vi "PSUN8731A-CTRLv2.vi"() -> ()   [LabVIEW 2017]
uses:
  Keysight N8731A conversion/Keysight N8900 Series.lvlib
panel:
  in  "Visible":bool
  in  "End Program":bool
  in  "PSU\nVoltage":bool caption="Keithley\nVoltage"
  in  "Sweep":bool caption="Constant"
  in  "OV protection":bool
  in  "Filename":string caption="Leave empty to discard data."
  out "Sweeping Back":bool
  in  "OC protection":bool
  in  "OV Value (10V)":dbl=10.0 min=0.5 max=10.0
  in  "Start Sweep":bool
  in  "Stop Sweep":bool
  in  "Sweep Controller":enum32{"CC Sweep", "Free Control", "VC Sweep"}(tab)
  in  "Voltage Limit [V]":dbl=8.0 min=0.0 max=8.0
  in  "Time Delay [s]":dbl=0.15
  in  "Step Size [A]":dbl=5.0 min=0.0 max=400.0
  in  "Start Current [A]":dbl min=0.0 max=400.0
  in  "End Current [A]":dbl=50.0 min=0.0 max=400.0
  out "Approx Run Time [min]":dbl
  in  "Current Limit [A]":dbl=150.0 min=0.0 max=400.0
  in  "Time Delay [s]":dbl=0.15 min=0.0
  in  "Step Size [mV]":dbl=10.0 min=0.0
  in  "Start Voltage [V]":dbl min=0.0 max=8.0
  in  "End Voltage[V]":dbl=0.1 min=0.0 max=8.0
  out "Approx Run Time [min]":dbl
  in  "VISA resource name":refnum<visa-resource-name>
  out "XY Graph":cluster{dbl[], dbl[]}(graph)
  # "Requires the subVIs in the \"Controller subVIs\" folder to function."
  # "\"Stop Sweep\" will immediately begin sweeping back to 0."
  # "Correct VISA option: TCPIP0::A-N8731A-8956R.local::inst0::INSTR\nfor lab computer or N8731APSU on the EPR computer."
  # "Sweep type will be automatically chosen according to open tab"
  # "Parameters may be\nedited before starting\nsweep"
  # "In case of errors, first check whether OVP or\nOCP has been triggered, or if parameters are \noutside allowed range. Currently leading causes\nof crashes."
  # "OCP not functional with CC\nsweeps, reason thus far unknown.\nSolution: disable OCP if safe."
  # "Data will be saved in .txt format, further analysis should be done on a\nseparate platform such as Gnuplot."
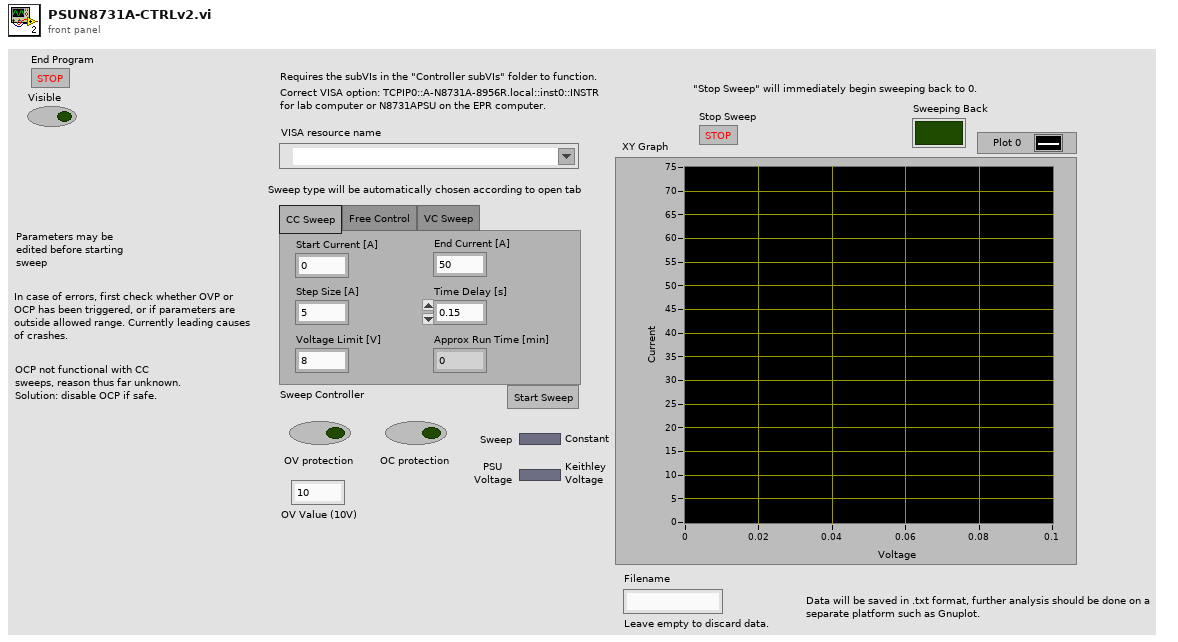
[diagram p1: front panel]
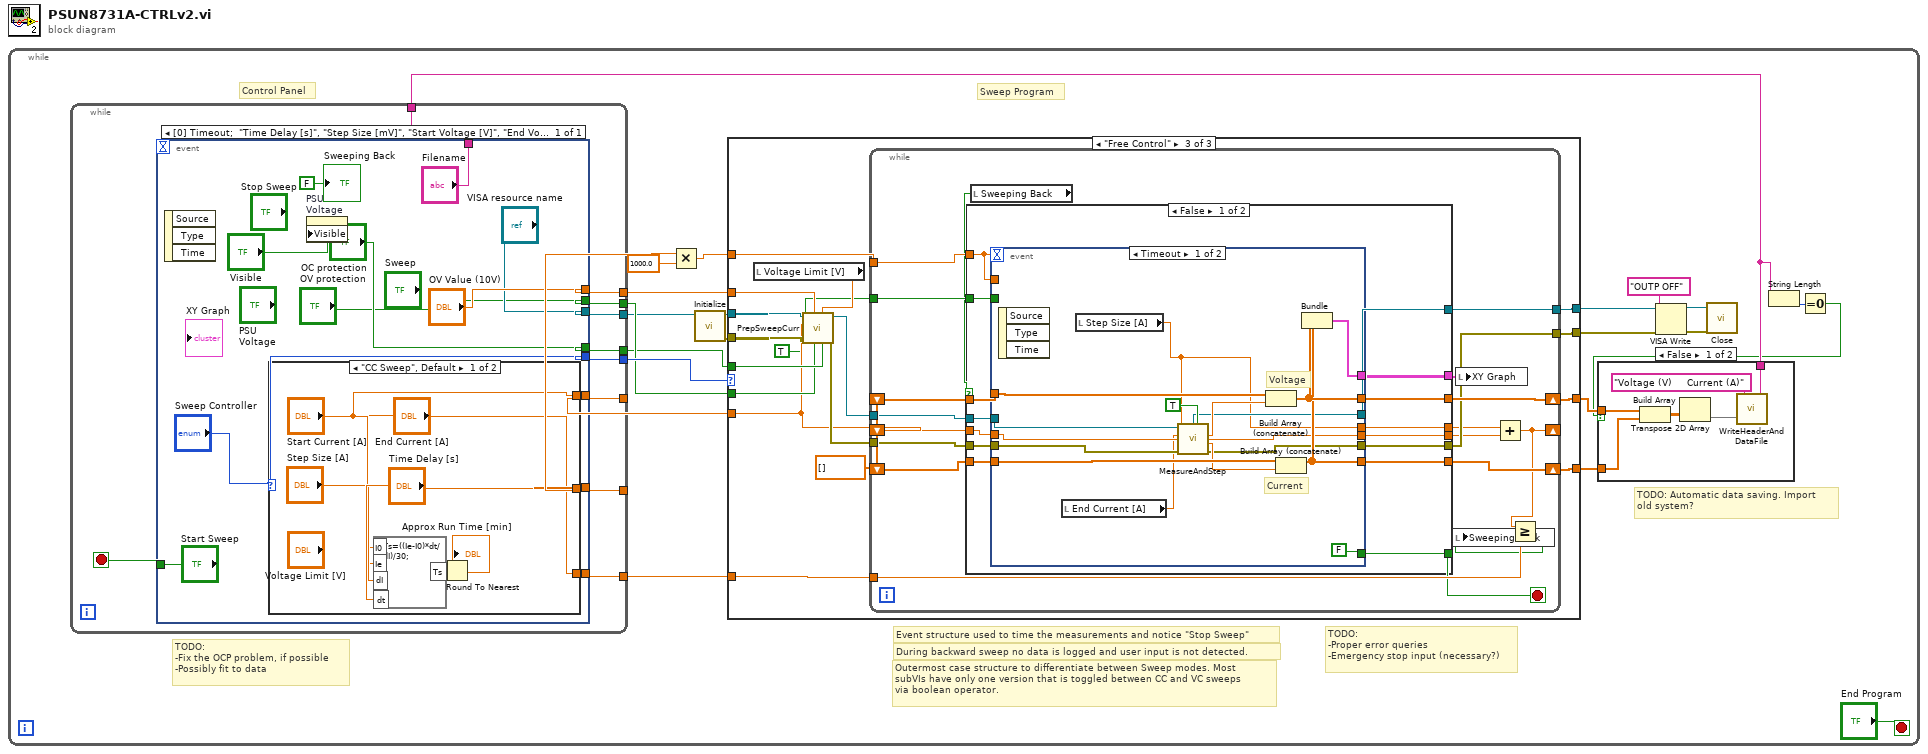
[diagram p0: block diagram]
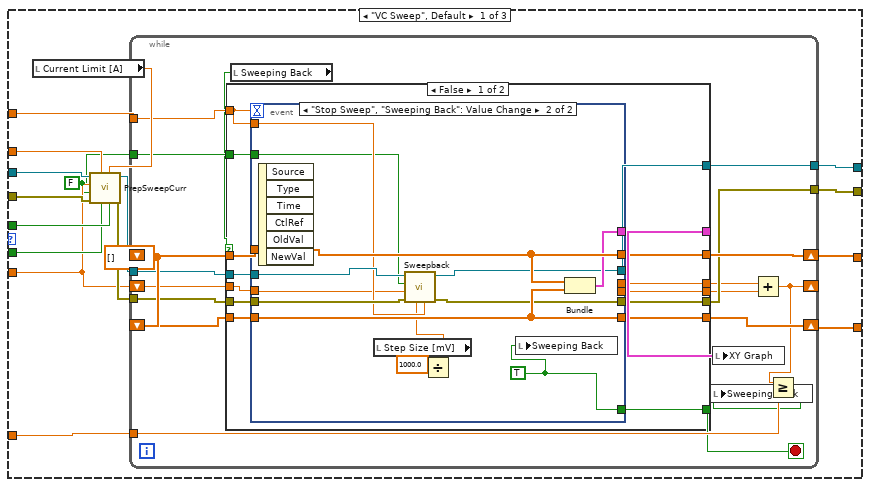
[diagram p3: hidden frame]
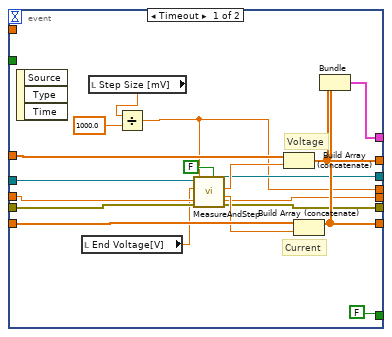
[diagram p4: hidden frame]
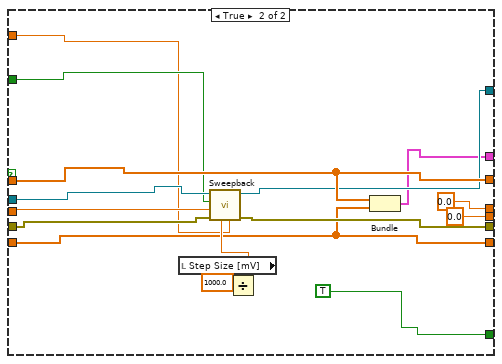
[diagram p5: hidden frame]
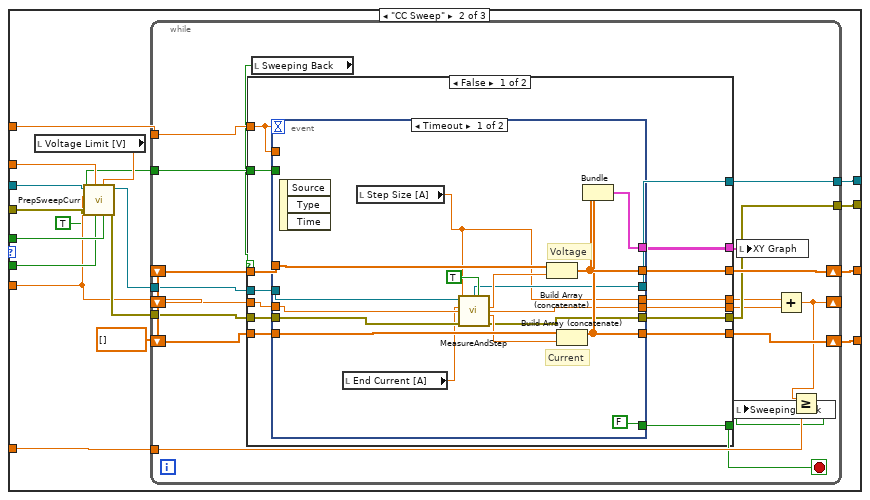
[diagram p6: hidden frame]
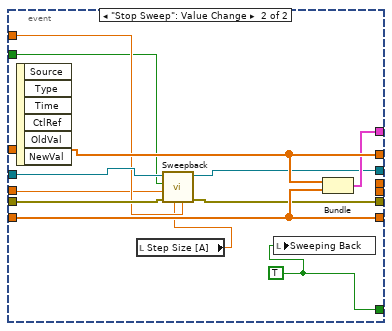
[diagram p7: hidden frame]
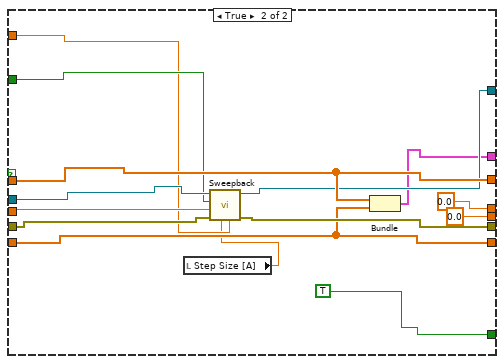
[diagram p8: hidden frame]
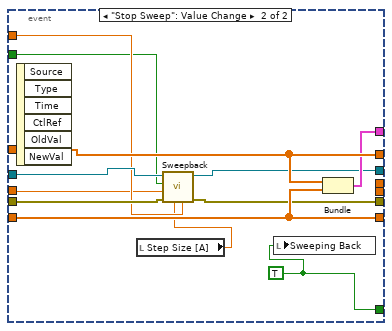
[diagram p9: hidden frame]
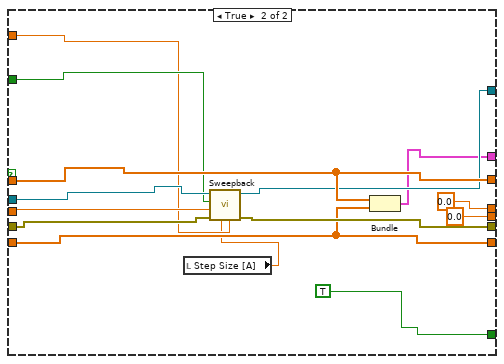
[diagram p10: hidden frame]
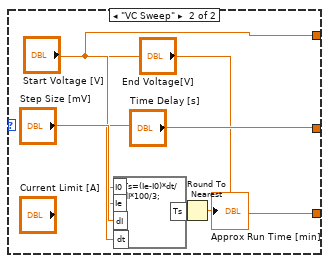
[diagram p11: hidden frame]
diagram:
  n1 = while {
    stop <- "End Program" stop-if-true
    # "TODO: \n-Proper error queries\n-Emergency stop input (necessary?)"
    # "TODO: Automatic data saving. Import\nold system?"
    # "TODO: \n-Fix the OCP problem, if possible\n-Possibly fit to data"
    # "Outermost case structure to differentiate between Sweep modes. Most\nsubVIs have only one version that is toggled between CC and VC sweeps\nvia boolean operator."
    # "During backward sweep no data is logged and user input is not detected."
    # "Event structure used to time the measurements and notice \"Stop Sweep\""
    # "Sweep Program"
    # "Control Panel"
    n2 = while {
      tunnel: [w324] -> w11
      tunnel: [w322] -> w23
      tunnel: [w321] -> w22
      tunnel: [w320] -> w8
      tunnel: [w315] -> w19
      tunnel: [w319] -> w18
      tunnel: [w318] -> w17
      tunnel: [w317] -> w7
      tunnel: [w316] -> w4
      stop <- w323 stop-if-true
      n3 = event shown="[0] Timeout;  \"Time Delay [s]\", \"Step Size [mV]\", \"Start Voltage [V]\", \"End Voltage[V]\", \"XY Graph\", \"VISA resource name\", \"Sweep Controller\", \"End Current [A]\", \"Stop Sweep\", \"Start Current [A]\", \"Step Size [A]\", \"Time Delay [s]\", \"Current Limit [A]\", \"Voltage Limit [V]\", \"Start Sweep\", \"Approx Run Time [min]\", \"Approx Run Time [min]\", \"OV Value (10V)\", \"OC protection\", \"Sweeping Back\", \"Filename\", \"OV protection\", \"PSU Voltage\": Value Change" {
        selector: _ -> [_]
        dyn-events: _ -> [_]
        timeout: _ -> [_]
        tunnel: [w336] -> w324
        tunnel: ["Start Sweep"] -> w323
        tunnel: [w334] -> w322
        tunnel: ["Sweep Controller"] -> w321
        tunnel: ["OC protection"] -> w320
        tunnel: ["OV Value (10V)"] -> w319
        tunnel: [w330] -> w318
        tunnel: ["VISA resource name"] -> w317
        tunnel: ["Filename"] -> w316
        tunnel: ["OV protection"] -> w315
        event Timeout; "Time Delay [s]", "Step Size [mV]", "Start Voltage [V]", "End Voltage[V]", "XY Graph", "VISA resource name", "Sweep Controller", "End Current [A]", "Stop Sweep", "Start Current [A]", "Step Size [A]", "Time Delay [s]", "Current Limit [A]", "Voltage Limit [V]", "Start Sweep", "Approx Run Time [min]", "Approx Run Time [min]", "OV Value (10V)", "OC protection", "Sweeping Back", "Filename", "OV protection", "PSU\nVoltage": Value Change {
          n4 = event-data() -> ()  [unwired: 1 in, 3 out]
          n5 = case shown="\"CC Sweep\", Default" "Sweep Controller" {
            tunnel: ["Time Delay [s]" "Time Delay [s]"] -> w336
            tunnel: ["Start Current [A]" "Start Voltage [V]"] -> w334
            tunnel: ["End Current [A]" "End Voltage[V]"] -> w330
            frame "CC Sweep", Default {
              n6 = formula code="Ts=((Ie-I0)*dt/dI)/30;"("I0"="Start Current [A]", "Ie"="End Current [A]", "dI"="Step Size [A]", "dt"="Time Delay [s]") -> ("Ts"=w340:dbl)
              n7 = Round To Nearest(number=w340) -> (nearest integer value=→"Approx Run Time [min]":dbl)
            }
            frame "VC Sweep" {
              n8 = formula code="Ts=(Ie-I0)*dt/dI*100/3;"("I0"="Start Voltage [V]", "Ie"="End Voltage[V]", "dI"="Step Size [mV]", "dt"="Time Delay [s]") -> ("Ts"=w346:dbl)
              n9 = Round To Nearest(number=w346) -> (nearest integer value=→"Approx Run Time [min]":dbl)
            }
          }
          n10 = property on="PSU\nVoltage" class="Bool (strict)"("Visible"="Visible") -> ()  [unwired: 2 in, 2 out]
          "Sweeping Back" <- FALSE ("Sweeping Back")
        }
      }
    }
    n11 = Multiply(x=w11, y=1000.0) -> (x*y=w10:dbl)
    n12 = call "Initialize.vi"("VISA resource name"=w7) -> ("error out"=w21:errorcluster, "VISA resource name out"=w20:refnum<visa-resource-name>)  [unwired: 9 in]
    n13 = case shown="\"Free Control\"" w22 {
      tunnel: w10 -> [w46 w145 w238]
      tunnel: w23 -> [w35 w134 w227]
      tunnel: w21 -> [w45 w144 w237]
      tunnel: w20 -> [w44 w143 w236]
      tunnel: [w41 w140 w233] -> w15
      tunnel: [w40 w139 w232] -> w16
      tunnel: w8 -> [w39 w138 w231]
      tunnel: w19 -> [w38 w137 w230]
      tunnel: w18 -> [w37 w136 w229]
      tunnel: w17 -> [w34 w133 w226]
      tunnel: [w31 w130 w223] -> w6
      tunnel: [w30 w129 w222] -> w5
      frame "VC Sweep", Default {
        w32 = dbl[] []
        w33 = FALSE ("CC (1)/VC (0)")
        n14 = local read "Current Limit [A]"() -> (w36:dbl)
        n15 = call "PrepSweepCurr.vi"("OC protection"=w39, "Voltage/Current Limit (0V/A)"=w36, "OV protection"=w38, "OV Value (10V)"=w37, "error in (no error)"=w45, "CC (1)/VC (0)"=w33, "Start Current/Voltage (0 A/V)"=w35, "VISA resource name"=w44) -> ("error out"=w42:errorcluster, "VISA resource name out"=w43:refnum<visa-resource-name>)  [unwired: 2 in]
        n16 = while {
          tunnel: w46 -> [w52]
          shift-right: [w65] -> w31
          shift-left: w32 -> [w63]
          shift-right: [w64] -> w30
          shift-left: w32 -> [w62]
          tunnel: w43 -> [w61]
          tunnel: w42 -> [w60]
          tunnel: [w59] -> w41
          tunnel: [w58] -> w40
          shift-right: [w55] -> _
          shift-left: w35 -> [w50]
          tunnel: w34 -> [w53]
          tunnel: w33 -> [w51]
          stop <- w49 stop-if-true
          n17 = local read "Sweeping Back"() -> (w48:bool)
          n18 = case shown="False" w48 {
            tunnel: [w80 w121] -> w65
            tunnel: [w79 w117] -> w64
            tunnel: w63 -> [w78 w121]
            tunnel: w62 -> [w77 w117]
            tunnel: w61 -> [w76 w122]
            tunnel: w60 -> [w75 w124]
            tunnel: [w74 w120] -> w59
            tunnel: [w73 w118] -> w58
            tunnel: [w72 0.0 ("Start Voltage [V]")] -> w57
            tunnel: [w71 w119] -> w56
            tunnel: [w70 0.0] -> w54
            tunnel: w52 -> [w69 w115]
            tunnel: w51 -> [w68 w116]
            tunnel: w50 -> [w67 w123]
            tunnel: [w66 TRUE] -> w49
            frame False {
              n19 = event shown="[1] \"Stop Sweep\", \"Sweeping Back\": Value Change" {
                selector: _ -> [_ _]
                dyn-events: _ -> [_ _]
                timeout: w69 -> [_ _]
                tunnel: [w98 w110] -> w71
                tunnel: [w97 w112] -> w80
                tunnel: [w96 w111] -> w79
                tunnel: w78 -> [w95 w112]
                tunnel: w77 -> [w94 w111]
                tunnel: [FALSE w99] -> w66
                tunnel: w76 -> [w87 w109]
                tunnel: w75 -> [w86 w107]
                tunnel: [w88 w106] -> w73
                tunnel: [w89 w108] -> w74
                tunnel: w67 -> [w85 w100]
                tunnel: [w85 _] -> w72
                tunnel: [w82 _] -> w70
                tunnel: w69 -> [_ w105]
                tunnel: w68 -> [_ w101]
                event Timeout {
                  # "Current"
                  # "Voltage"
                  n20 = event-data() -> ()  [unwired: 1 in, 3 out]
                  n21 = local read "End Voltage[V]"() -> (w81:dbl)
                  n22 = local read "Step Size [mV]"() -> (w84:dbl)
                  n23 = Divide(x=w84, y=1000.0) -> (x/y=w82:dbl)
                  n24 = call "MeasureAndStep.vi"("CC (1)/VC (0)"=FALSE ("Current (1)/Voltage (0)"), "Last Current/Voltage Value (0 A/V)"=w85, "error in (no error)"=w86, "Current/Voltage Step (0 A/V)"=w82, "End Current/Voltage [A/V]"=w81, "VISA resource name"=w87) -> ("error out"=w88:errorcluster, "CURR"=w92:dbl, "VOLT"=w93:dbl, "VISA resource name out"=w89:refnum<visa-resource-name>)  [unwired: 2 in]
                  n25 = Build Array (concatenate)(w95, w93) -> (w97:dbl[])
                  n26 = Build Array (concatenate)(w94, w92) -> (w96:dbl[])
                  n27 = Bundle(w97, w96) -> (w98:cluster{dbl[], dbl[]})  [unwired: 1 in]
                }
                event "Stop Sweep", "Sweeping Back": Value Change {
                  w99 = TRUE
                  n28 = event-data() -> ()  [unwired: 1 in, 6 out]
                  n29 = local read "Step Size [mV]"() -> (w104:dbl)
                  n30 = Divide(x=w104, y=1000.0) -> (x/y=w102:dbl)
                  n31 = call "Sweepback.vi"("Time Between Steps [ms]"=w105, "Step Size [A/V]"=w102, "error in (no error)"=w107, "Max reached Current/Voltage [A/V]"=w100, "CC (1)/VC (0)"=w101, "VISA resource name"=w109) -> ("error out"=w106:errorcluster, "VISA resource name out"=w108:refnum<visa-resource-name>)  [unwired: 4 in]
                  n32 = local write "Sweeping Back"(w99) -> ()
                  n33 = Bundle(w112, w111) -> (w110:cluster{dbl[], dbl[]})  [unwired: 1 in]
                }
              }
            }
            frame True {
              n34 = local read "Step Size [mV]"() -> (w128:dbl)
              n35 = Divide(x=w128, y=1000.0) -> (x/y=w126:dbl)
              n36 = call "Sweepback.vi"("Time Between Steps [ms]"=w115, "Step Size [A/V]"=w126, "error in (no error)"=w124, "Max reached Current/Voltage [A/V]"=w123, "CC (1)/VC (0)"=w116, "VISA resource name"=w122) -> ("error out"=w118:errorcluster, "VISA resource name out"=w120:refnum<visa-resource-name>)  [unwired: 4 in]
              n37 = Bundle(w121, w117) -> (w119:cluster{dbl[], dbl[]})  [unwired: 1 in]
            }
          }
          n38 = local write "XY Graph"(w56) -> ()
          n39 = Add(x=w54, y=w57) -> (x+y=w55:dbl)
          n40 = Greater Or Equal?(x=w55, y=w53) -> (x >= y?=w47:bool)
          n41 = local write "Sweeping Back"(w47) -> ()
        }
      }
      frame "CC Sweep" {
        w131 = dbl[] []
        w132 = TRUE ("CC (1)/VC (0)")
        n42 = local read "Voltage Limit [V]"() -> (w135:dbl)
        n43 = call "PrepSweepCurr.vi"("OC protection"=w138, "Voltage/Current Limit (0V/A)"=w135, "OV protection"=w137, "OV Value (10V)"=w136, "error in (no error)"=w144, "CC (1)/VC (0)"=w132, "Start Current/Voltage (0 A/V)"=w134, "VISA resource name"=w143) -> ("error out"=w141:errorcluster, "VISA resource name out"=w142:refnum<visa-resource-name>)  [unwired: 2 in]
        n44 = while {
          tunnel: w145 -> [w151]
          shift-right: [w164] -> w130
          shift-left: w131 -> [w162]
          shift-right: [w163] -> w129
          shift-left: w131 -> [w161]
          tunnel: w142 -> [w160]
          tunnel: w141 -> [w159]
          tunnel: [w158] -> w140
          tunnel: [w157] -> w139
          shift-right: [w154] -> _
          shift-left: w134 -> [w149]
          tunnel: w133 -> [w152]
          tunnel: w132 -> [w150]
          stop <- w148 stop-if-true
          n45 = local read "Sweeping Back"() -> (w147:bool)
          n46 = case shown="False" w147 {
            tunnel: [w179 w217] -> w164
            tunnel: [w178 w213] -> w163
            tunnel: w162 -> [w177 w217]
            tunnel: w161 -> [w176 w213]
            tunnel: w160 -> [w175 w218]
            tunnel: w159 -> [w174 w220]
            tunnel: [w173 w216] -> w158
            tunnel: [w172 w214] -> w157
            tunnel: [w171 0.0 ("Start Voltage [V]")] -> w156
            tunnel: [w170 w215] -> w155
            tunnel: [w169 0.0] -> w153
            tunnel: w151 -> [w165 w211]
            tunnel: w150 -> [w168 w212]
            tunnel: w149 -> [w167 w219]
            tunnel: [w166 TRUE] -> w148
            frame False {
              n47 = event shown="[0] Timeout" {
                selector: _ -> [_ _]
                dyn-events: _ -> [_ _]
                timeout: w165 -> [_ _]
                tunnel: [w195 w205] -> w170
                tunnel: [w194 w207] -> w179
                tunnel: [w193 w206] -> w178
                tunnel: w177 -> [w192 w207]
                tunnel: w176 -> [w191 w206]
                tunnel: [FALSE w197] -> w166
                tunnel: w175 -> [w184 w204]
                tunnel: w174 -> [w183 w202]
                tunnel: [w185 w201] -> w172
                tunnel: [w186 w203] -> w173
                tunnel: w167 -> [w182 w198]
                tunnel: [w182 _] -> w171
                tunnel: [w181 _] -> w169
                tunnel: w165 -> [_ w200]
                tunnel: w168 -> [_ w199]
                event Timeout {
                  # "Current"
                  # "Voltage"
                  n48 = event-data() -> ()  [unwired: 1 in, 3 out]
                  n49 = local read "End Current [A]"() -> (w180:dbl)
                  n50 = local read "Step Size [A]"() -> (w181:dbl)
                  n51 = call "MeasureAndStep.vi"("CC (1)/VC (0)"=TRUE ("Current (1)/Voltage (0)"), "Last Current/Voltage Value (0 A/V)"=w182, "error in (no error)"=w183, "Current/Voltage Step (0 A/V)"=w181, "End Current/Voltage [A/V]"=w180, "VISA resource name"=w184) -> ("error out"=w185:errorcluster, "CURR"=w189:dbl, "VOLT"=w190:dbl, "VISA resource name out"=w186:refnum<visa-resource-name>)  [unwired: 2 in]
                  n52 = Build Array (concatenate)(w192, w190) -> (w194:dbl[])
                  n53 = Build Array (concatenate)(w191, w189) -> (w193:dbl[])
                  n54 = Bundle(w194, w193) -> (w195:cluster{dbl[], dbl[]})  [unwired: 1 in]
                }
                event "Stop Sweep": Value Change {
                  w197 = TRUE
                  n55 = event-data() -> ()  [unwired: 1 in, 6 out]
                  n56 = local read "Step Size [A]"() -> (w196:dbl)
                  n57 = call "Sweepback.vi"("Time Between Steps [ms]"=w200, "Step Size [A/V]"=w196, "error in (no error)"=w202, "Max reached Current/Voltage [A/V]"=w198, "CC (1)/VC (0)"=w199, "VISA resource name"=w204) -> ("error out"=w201:errorcluster, "VISA resource name out"=w203:refnum<visa-resource-name>)  [unwired: 4 in]
                  n58 = local write "Sweeping Back"(w197) -> ()
                  n59 = Bundle(w207, w206) -> (w205:cluster{dbl[], dbl[]})  [unwired: 1 in]
                }
              }
            }
            frame True {
              n60 = local read "Step Size [A]"() -> (w208:dbl)
              n61 = call "Sweepback.vi"("Time Between Steps [ms]"=w211, "Step Size [A/V]"=w208, "error in (no error)"=w220, "Max reached Current/Voltage [A/V]"=w219, "CC (1)/VC (0)"=w212, "VISA resource name"=w218) -> ("error out"=w214:errorcluster, "VISA resource name out"=w216:refnum<visa-resource-name>)  [unwired: 4 in]
              n62 = Bundle(w217, w213) -> (w215:cluster{dbl[], dbl[]})  [unwired: 1 in]
            }
          }
          n63 = local write "XY Graph"(w155) -> ()
          n64 = Add(x=w153, y=w156) -> (x+y=w154:dbl)
          n65 = Greater Or Equal?(x=w154, y=w152) -> (x >= y?=w146:bool)
          n66 = local write "Sweeping Back"(w146) -> ()
        }
      }
      frame "Free Control" {
        w224 = dbl[] []
        w225 = TRUE ("CC (1)/VC (0)")
        n67 = local read "Voltage Limit [V]"() -> (w228:dbl)
        n68 = call "PrepSweepCurr.vi"("OC protection"=w231, "Voltage/Current Limit (0V/A)"=w228, "OV protection"=w230, "OV Value (10V)"=w229, "error in (no error)"=w237, "CC (1)/VC (0)"=w225, "Start Current/Voltage (0 A/V)"=w227, "VISA resource name"=w236) -> ("error out"=w234:errorcluster, "VISA resource name out"=w235:refnum<visa-resource-name>)  [unwired: 2 in]
        n69 = while {
          tunnel: w238 -> [w244]
          shift-right: [w257] -> w223
          shift-left: w224 -> [w255]
          shift-right: [w256] -> w222
          shift-left: w224 -> [w254]
          tunnel: w235 -> [w253]
          tunnel: w234 -> [w252]
          tunnel: [w251] -> w233
          tunnel: [w250] -> w232
          shift-right: [w247] -> _
          shift-left: w227 -> [w242]
          tunnel: w226 -> [w245]
          tunnel: w225 -> [w243]
          stop <- w241 stop-if-true
          n70 = local read "Sweeping Back"() -> (w240:bool)
          n71 = case shown="False" w240 {
            tunnel: [w272 w310] -> w257
            tunnel: [w271 w306] -> w256
            tunnel: w255 -> [w270 w310]
            tunnel: w254 -> [w269 w306]
            tunnel: w253 -> [w268 w311]
            tunnel: w252 -> [w267 w313]
            tunnel: [w266 w309] -> w251
            tunnel: [w265 w307] -> w250
            tunnel: [w264 0.0 ("Start Voltage [V]")] -> w249
            tunnel: [w263 w308] -> w248
            tunnel: [w262 0.0] -> w246
            tunnel: w244 -> [w258 w304]
            tunnel: w243 -> [w261 w305]
            tunnel: w242 -> [w260 w312]
            tunnel: [w259 TRUE] -> w241
            frame False {
              n72 = event shown="[0] Timeout" {
                selector: _ -> [_ _]
                dyn-events: _ -> [_ _]
                timeout: w258 -> [_ _]
                tunnel: [w288 w298] -> w263
                tunnel: [w287 w300] -> w272
                tunnel: [w286 w299] -> w271
                tunnel: w270 -> [w285 w300]
                tunnel: w269 -> [w284 w299]
                tunnel: [FALSE w290] -> w259
                tunnel: w268 -> [w277 w297]
                tunnel: w267 -> [w276 w295]
                tunnel: [w278 w294] -> w265
                tunnel: [w279 w296] -> w266
                tunnel: w260 -> [w275 w291]
                tunnel: [w275 _] -> w264
                tunnel: [w274 _] -> w262
                tunnel: w258 -> [_ w293]
                tunnel: w261 -> [_ w292]
                event Timeout {
                  # "Current"
                  # "Voltage"
                  n73 = event-data() -> ()  [unwired: 1 in, 3 out]
                  n74 = local read "End Current [A]"() -> (w273:dbl)
                  n75 = local read "Step Size [A]"() -> (w274:dbl)
                  n76 = call "MeasureAndStep.vi"("CC (1)/VC (0)"=TRUE ("Current (1)/Voltage (0)"), "Last Current/Voltage Value (0 A/V)"=w275, "error in (no error)"=w276, "Current/Voltage Step (0 A/V)"=w274, "End Current/Voltage [A/V]"=w273, "VISA resource name"=w277) -> ("error out"=w278:errorcluster, "CURR"=w282:dbl, "VOLT"=w283:dbl, "VISA resource name out"=w279:refnum<visa-resource-name>)  [unwired: 2 in]
                  n77 = Build Array (concatenate)(w285, w283) -> (w287:dbl[])
                  n78 = Build Array (concatenate)(w284, w282) -> (w286:dbl[])
                  n79 = Bundle(w287, w286) -> (w288:cluster{dbl[], dbl[]})  [unwired: 1 in]
                }
                event "Stop Sweep": Value Change {
                  w290 = TRUE
                  n80 = event-data() -> ()  [unwired: 1 in, 6 out]
                  n81 = local read "Step Size [A]"() -> (w289:dbl)
                  n82 = call "Sweepback.vi"("Time Between Steps [ms]"=w293, "Step Size [A/V]"=w289, "error in (no error)"=w295, "Max reached Current/Voltage [A/V]"=w291, "CC (1)/VC (0)"=w292, "VISA resource name"=w297) -> ("error out"=w294:errorcluster, "VISA resource name out"=w296:refnum<visa-resource-name>)  [unwired: 4 in]
                  n83 = local write "Sweeping Back"(w290) -> ()
                  n84 = Bundle(w300, w299) -> (w298:cluster{dbl[], dbl[]})  [unwired: 1 in]
                }
              }
            }
            frame True {
              n85 = local read "Step Size [A]"() -> (w301:dbl)
              n86 = call "Sweepback.vi"("Time Between Steps [ms]"=w304, "Step Size [A/V]"=w301, "error in (no error)"=w313, "Max reached Current/Voltage [A/V]"=w312, "CC (1)/VC (0)"=w305, "VISA resource name"=w311) -> ("error out"=w307:errorcluster, "VISA resource name out"=w309:refnum<visa-resource-name>)  [unwired: 4 in]
              n87 = Bundle(w310, w306) -> (w308:cluster{dbl[], dbl[]})  [unwired: 1 in]
            }
          }
          n88 = local write "XY Graph"(w248) -> ()
          n89 = Add(x=w246, y=w249) -> (x+y=w247:dbl)
          n90 = Greater Or Equal?(x=w247, y=w245) -> (x >= y?=w239:bool)
          n91 = local write "Sweeping Back"(w239) -> ()
        }
      }
    }
    n92 = VISA Write(VISA resource name=w15, write buffer="OUTP OFF", error in (no error)=w16) -> (VISA resource name out=w12:refnum<visa-resource-name>, error out=w13:errorcluster)  [unwired: 1 out]
    n93 = call "Close.vi"("error in (no error)"=w13, "VISA resource name"=w12) -> ()  [unwired: 9 in, 1 out]
    n94 = String Length(string=w4) -> (length=w3:i32)
    n95 = Equal To 0?(x=w3) -> (x = 0?=w2:bool)
    n96 = case shown="False" w2 {
      tunnel: w6 -> [w29 _]
      tunnel: w5 -> [w28 _]
      tunnel: w4 -> [w24 _]
      frame False {
        n97 = Build Array(w29, w28) -> (w27:dbl[][])
        n98 = Transpose 2D Array(2D array=w27) -> (transposed array=w26:dbl[][])
        n99 = call "WriteHeaderAndDataFile.vi"("filename"=w24, "Array"=w26, "Header"="Voltage (V)     Current (A)") -> ()
      }
      frame True {
      }
    }
  }
